vi "Merge Data.vi"(8 "error in":errorcluster, 10 "Analyzed":refnum<class "Instrument.lvclass">, 11 "Acquired":refnum<class "nCRD.lvclass">) -> (0 "error out":errorcluster, 3 "nCRD out":refnum<class "nCRD.lvclass">)   [LabVIEW 2013, in "nCRD.lvclass"]
doc: "The VI Merge Data is used strictly here to merge the serial data with the rest of the data. THIS VI WILL BE NO LONGER NECESSARY WHEN ISSUES RELATING TO RT EXE ARE FIXED!!"
uses:
  nCRD.lvclass
  Reusable/Instrument/Instrument.lvclass
  Reusable/CRDS/Main/CRDS.lvclass
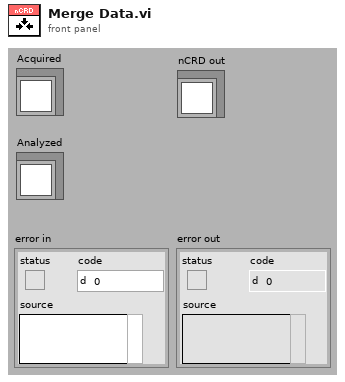
[diagram p1: front panel]
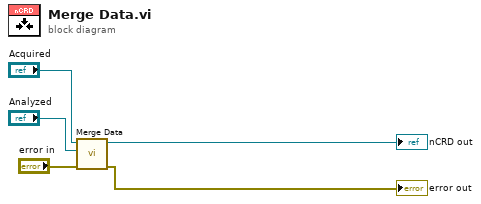
[diagram p0: block diagram]
diagram:
  n1 = call-parent "Merge Data.vi"("error in"="error in", "Analyzed"="Analyzed", "Acquired"="Acquired") -> ("error out"=→"error out":errorcluster, "CRDS out"=→"nCRD out":refnum<class "nCRD.lvclass">)  [unwired: 7 in]
